vi "Destroy.vi"(8 "ErrorIn":errorcluster, 11 "ReferenceIn":refnum<class "JSONTextViewer.lvclass">) -> (0 "ErrorOut":errorcluster, 3 "ReferenceOut":refnum<class "JSONTextViewer.lvclass">)   [LabVIEW 2021, in "JSONTextViewer.lvlib" / "JSONTextViewer.lvclass"]
uses:
  JSONTextViewer.lvclass
  .Externals/Library_TAF_ApplicationFramework/TAFBaseGUI/TAFBaseGUI.lvclass
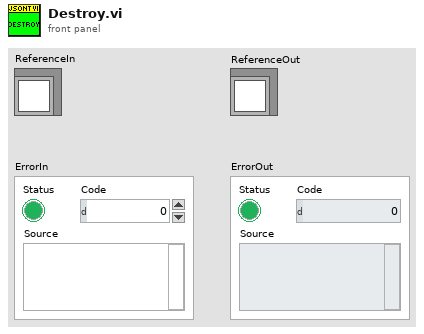
[diagram p1: front panel]
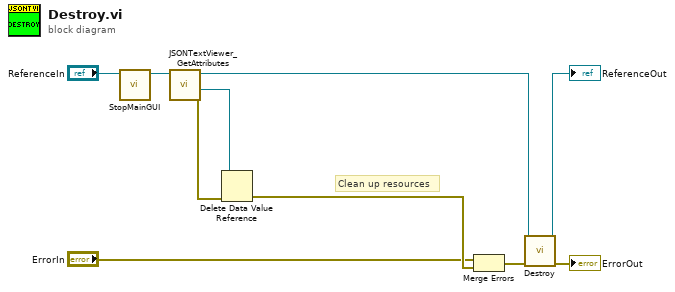
[diagram p0: block diagram]
diagram:
  # "Clean up resources"
  n1 = call "StopMainGUI.vi"("ReferenceIn"="ReferenceIn") -> ("ReferenceOut"=w3:refnum<class "JSONTextViewer.lvclass">)  [unwired: 9 in, 1 out]
  n2 = call "JSONTextViewer_GetAttributes.vi"("ReferenceIn"=w3) -> ("ErrorOut"=w10:errorcluster, "DataRef"=w5:refnum<data-value>, "ReferenceOut"=w2:refnum<class "JSONTextViewer.lvclass">)  [unwired: 7 in, 1 out]
  n3 = Delete Data Value Reference(data value reference=w5, error in=w10) -> (error out=w9:errorcluster)  [unwired: 1 out]
  n4 = Merge Errors("ErrorIn", w9) -> (w7:errorcluster)
  n5 = call-parent "Destroy.vi"("ErrorIn"=w7, "ReferenceIn"=w2) -> ("ErrorOut"=→"ErrorOut":errorcluster, "ReferenceOut"=→"ReferenceOut":refnum<class "JSONTextViewer.lvclass">)  [unwired: 8 in]
